vi "LDA_Align_PN_orig.vi"(1 "Align Probe Using":enum16{"Green Beams", "Blue Beams"}(ring), 2 "Use Specification Beam Half-Angle":bool) -> (0 "Beam Data":T1={"Vg1 (Green 1 dir. vect.)"=[0.059117350659853476, -0.996541267827751, 0.05840068807144843], "Vg2  (Green 2 dir. vect.)"=[-0.05232536310393669, -0.9971561380468801, -0.054237373935992664], "Vb1 (Blue 1 dir. vect.)"=[-0.052923229613528855, -0.9969242065933935, 0.057803616456121795], "Vb2 (Blue 1 dir. vect.)"=[0.05971521716944564, -0.9967731992812374, -0.05364030232066602], "Porb (Orb XYZ posn. forced coplanar)"=[2201.0738225655555, -1199.3737231995547, 269.758310600838], "Porb (Orb XYZ posn. - allow skew)"=[2200.796256301178, -1199.3740953152687, 270.0329332816893], "Orb posn. uncertainty, +/- dx, dy, dz"=[0.13878313218879157, 0.00018605785703584843, 0.13731134042564008], "Vp (Actual Probe dir. vect)"=[0.003406702197773746, -0.9999920168246164, 0.0020882210543692924], "Yaw (deg)"=89.80480953887573, "Pitch (deg)"=0.11964634006213794, "In-Plane Roll (deg)"=45.305328966424156, "Beam Half Angle (deg)"=4.544091484248422, "B1 Close P11"=[0.0, 0.0, 0.0], "B1 Far P12"=[2158.01, -491.04, 229.28], "B2 Close P22"=[2158.01, -491.04, 229.28], "B2 Far P21"=[2158.01, -491.04, 229.28], "Projected Roll (deg)"=0.0, "Green Velocity Vector"=[0.0, 0.0, 0.0], "Blue Velocity Vector"=[0.0, 0.0, 0.0], "Probe is facing...."="-", "Calculation Method"=""} {"Vp (Actual Probe dir. vect)" format="%#_6f"; "Vg2  (Green 2 dir. vect.)" format="%#_6f"; "Vg1 (Green 1 dir. vect.)" format="%#_6f"})   [LabVIEW 2010]
uses:
  Controls/LDA_Beam_Cluster.ctl
  Controls/Tunnel_Coordinates.ctl
  Controls/User_Specific_mode.ctl
  Gen Trav/Trav_mode.ctl
  Globals/Trav_pos_global.vi
  Globals/LDA_meas_global_1.vi
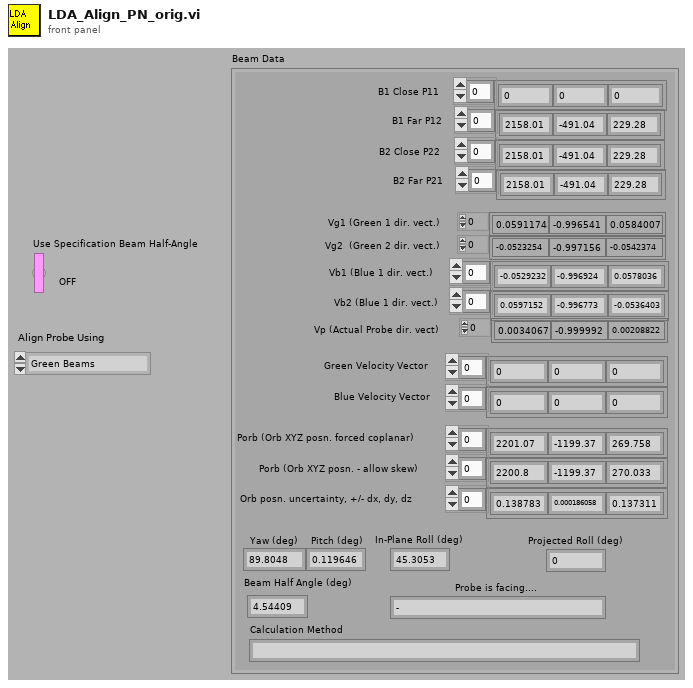
[diagram p1: front panel]
types:
  T1 = typedef "LDA_Beam_Cluster.ctl" = cluster{"Vg1 (Green 1 dir. vect.)":dbl[], "Vg2  (Green 2 dir. vect.)":dbl[], "Vb1 (Blue 1 dir. vect.)":dbl[], "Vb2 (Blue 1 dir. vect.)":dbl[], "Porb (Orb XYZ posn. forced coplanar)":dbl[], "Porb (Orb XYZ posn. - allow skew)":dbl[], "Orb posn. uncertainty, +/- dx, dy, dz":dbl[], "Vp (Actual Probe dir. vect)":dbl[], "Yaw (deg)":dbl, "Pitch (deg)":dbl, "In-Plane Roll (deg)":dbl, "Beam Half Angle (deg)":dbl, "B1 Close P11":dbl[], "B1 Far P12":dbl[], "B2 Close P22":dbl[], "B2 Far P21":dbl[], "Projected Roll (deg)":dbl, "Green Velocity Vector":dbl[], "Blue Velocity Vector":dbl[], "Probe is facing....":string, "Calculation Method":string}
  T2 = typedef "Tunnel_Coordinates.ctl" = enum16{"Work in Tunnel Coordinates", "Work in Model Coordinates"}
  T3 = typedef "User_Specific_mode.ctl" = enum16{"Check VI only", "Run VI"}
  T4 = typedef "Trav_mode.ctl" = enum16{"Move traverse", "Read traverse position", "Teach Position"}
  T5 = enum16{"Load setup from excel file", "Save setup to excel file"}
  T6 = enum16{"Load From Excel File", "Save to Excel File"}
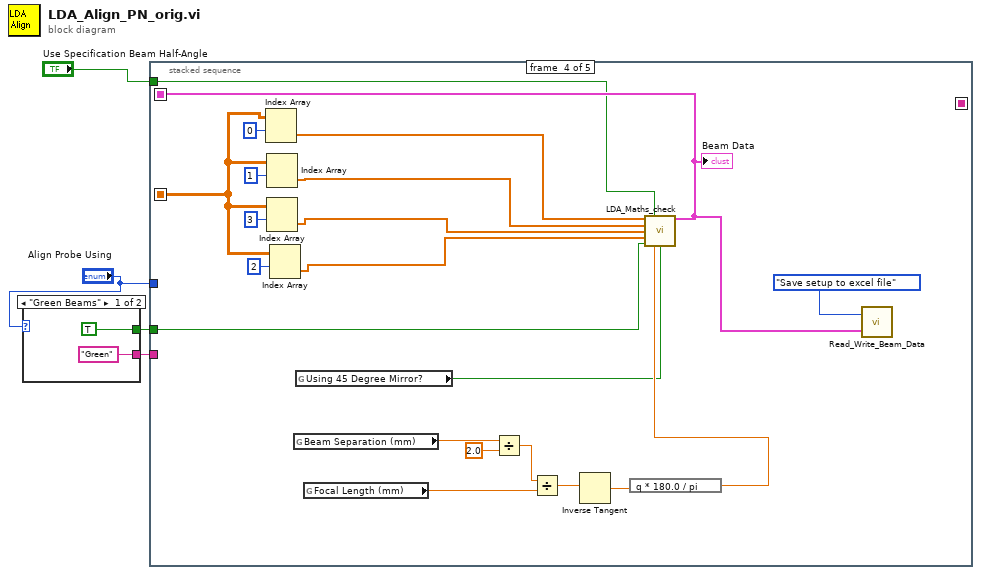
[diagram p0: block diagram]
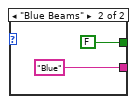
[diagram p2: hidden frame]
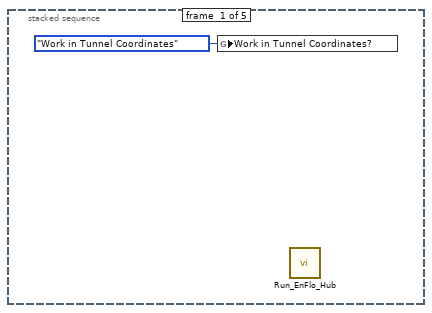
[diagram p3: hidden frame]
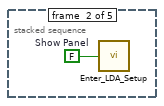
[diagram p4: hidden frame]
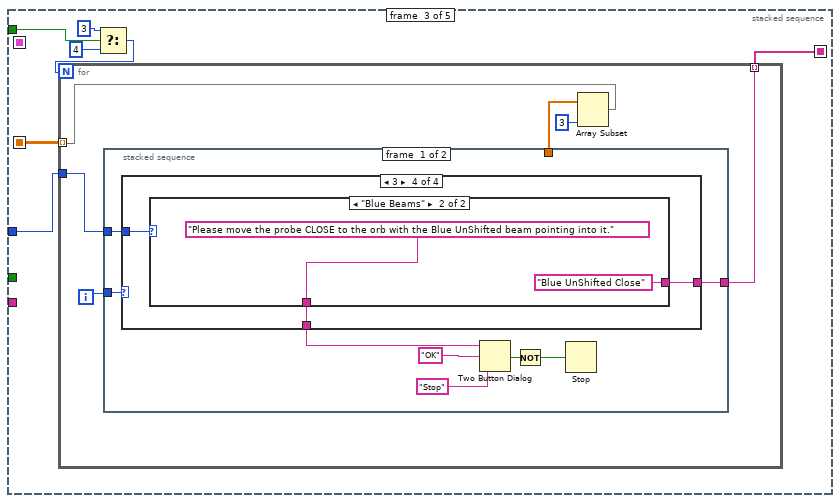
[diagram p5: hidden frame]
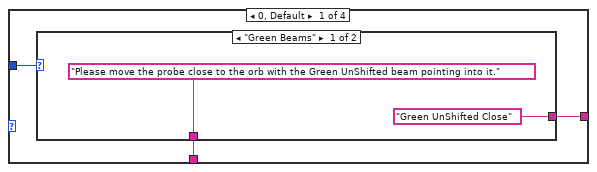
[diagram p6: hidden frame]
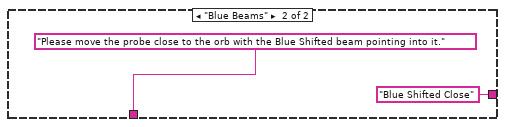
[diagram p7: hidden frame]
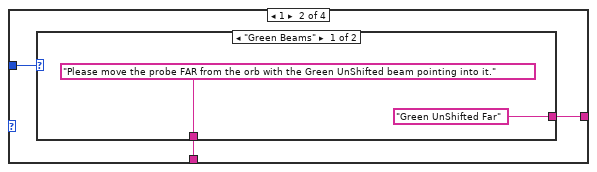
[diagram p8: hidden frame]
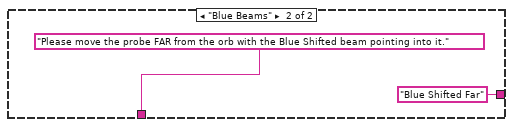
[diagram p9: hidden frame]
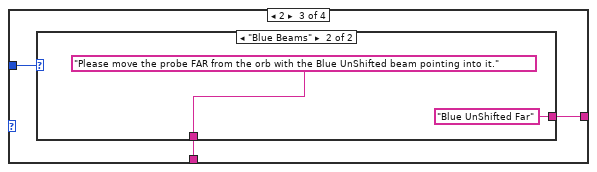
[diagram p10: hidden frame]
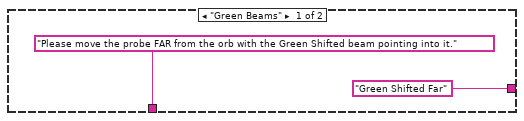
[diagram p11: hidden frame]
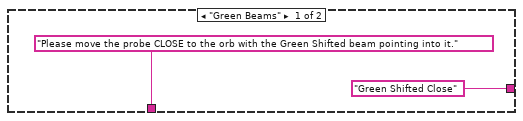
[diagram p12: hidden frame]
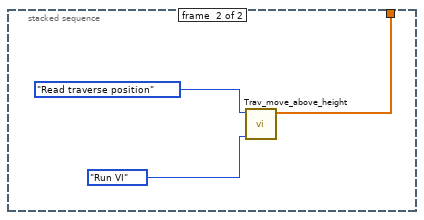
[diagram p13: hidden frame]
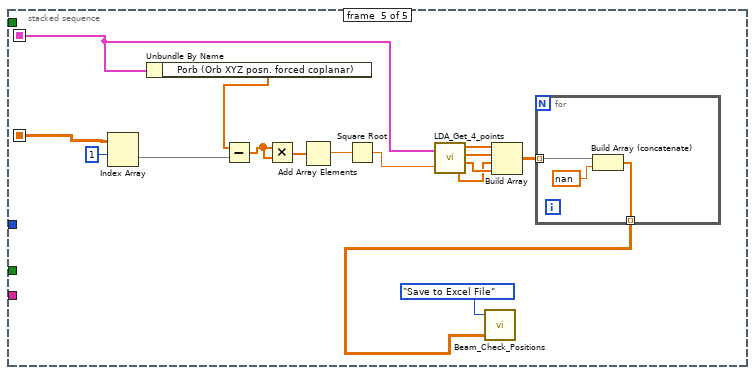
[diagram p14: hidden frame]
diagram:
  n1 = case shown="\"Green Beams\"" "Align Probe Using" {
    tunnel: [TRUE FALSE] -> w4
    tunnel: ["Green" "Blue"] -> w1
    frame "Green Beams" {
    }
    frame "Blue Beams" {
    }
  }
  n2 = stacked-sequence {
    seq-local: [_ _ _ w82 _] -> [_ _ _ _ w95]
    seq-local: [_ _ w11 _ _] -> [_ _ _ w64 w84]
    seq-local: [_ _ w12 _ _] -> [_ _ _ _ _]
    tunnel: w4 -> [_ _ _ w74 _]
    tunnel: "Use Specification Beam Half-Angle" -> [_ _ w16 w73 _]
    tunnel: "Align Probe Using" -> [_ _ w17 _ _]
    tunnel: w1 -> [_ _ _ _ _]
    frame #0 {
      n3 = global write "Trav_pos_global.vi" "Work in Tunnel Coordinates?"(Tunnel_Coordinates."Work in Tunnel Coordinates" ("Work in Tunnel Coordinates?")) -> ()
      n4 = call "Run_EnFlo_Hub.vi"() -> ()  [unwired: 8 in]
    }
    frame #1 {
      w10 = FALSE  # Show Panel
      n5 = call "Enter_LDA_Setup.vi"("Show Panel"=w10) -> ()
    }
    frame #2 {
      n6 = Select(t=3, s=w16, f=4) -> (s? t:f=w13:i32)
      n7 = for {
        N: w13 -> [_]
        tunnel: w17 -> [w23]
        tunnel: [w22] -> w12 mode=indexing
        tunnel: [w18] -> w11 mode=indexing
        i -> [w21]
        n8 = stacked-sequence {
          tunnel: [_ w60] -> w19
          tunnel: w23 -> [w30 _]
          tunnel: [w25 _] -> w22
          tunnel: w21 -> [w24 _]
          frame #0 {
            n9 = case shown="3" w24 {
              tunnel: [w34 w41 w48 w55] -> w31
              tunnel: w30 -> [w33 w40 w47 w54]
              tunnel: [w32 w39 w46 w53] -> w25
              frame 0, Default {
                n10 = case shown="\"Green Beams\"" w33 {
                  tunnel: ["Please move the probe close to the orb with the Green UnShifted beam pointing into it." ("message") "Please move the probe close to the orb with the Blue Shifted beam pointing into it." ("message")] -> w34
                  tunnel: ["Green UnShifted Close" "Blue Shifted Close"] -> w32
                  frame "Green Beams" {
                  }
                  frame "Blue Beams" {
                  }
                }
              }
              frame 1 {
                n11 = case shown="\"Green Beams\"" w40 {
                  tunnel: ["Please move the probe FAR from the orb with the Green UnShifted beam pointing into it." ("message") "Please move the probe FAR from the orb with the Blue Shifted beam pointing into it." ("message")] -> w41
                  tunnel: ["Green UnShifted Far" "Blue Shifted Far"] -> w39
                  frame "Green Beams" {
                  }
                  frame "Blue Beams" {
                  }
                }
              }
              frame 2 {
                n12 = case shown="\"Blue Beams\"" w47 {
                  tunnel: ["Please move the probe FAR from the orb with the Green Shifted beam pointing into it." ("message") "Please move the probe FAR from the orb with the Blue UnShifted beam pointing into it." ("message")] -> w48
                  tunnel: ["Green Shifted Far" "Blue UnShifted Far"] -> w46
                  frame "Green Beams" {
                  }
                  frame "Blue Beams" {
                  }
                }
              }
              frame 3 {
                n13 = case shown="\"Blue Beams\"" w54 {
                  tunnel: ["Please move the probe CLOSE to the orb with the Green Shifted beam pointing into it." ("message") "Please move the probe CLOSE to the orb with the Blue UnShifted beam pointing into it." ("message")] -> w55
                  tunnel: ["Green Shifted Close" "Blue UnShifted Close"] -> w53
                  frame "Green Beams" {
                  }
                  frame "Blue Beams" {
                  }
                }
              }
            }
            n14 = Two Button Dialog(message=w31, 1:"Stop" ("F button name (\"Cancel\")"), 2:"OK" ("T button name (\"OK\")")) -> (T button?=w27:bool)
            n15 = Not(x=w27) -> (.not. x?=w26:bool)
            n16 = Stop(stop? (T)=w26) -> ()
          }
          frame #1 {
            n17 = call "Trav_move_above_height.vi"("Simulate/Run"=User_Specific_mode."Run VI", "Mode"=Trav_mode."Read traverse position") -> ("Trav Position achieved"=w60:dbl[])  [unwired: 8 in, 1 out]
          }
        }
        n18 = Array Subset(array=w19, length=3) -> (w18:dbl[])  [unwired: 1 in]
      }
    }
    frame #3 {
      n19 = Index Array(array=w64, index (row)=0) -> (element=w68:dbl[])  [unwired: 1 in]
      n20 = Index Array(array=w64, index (row)=1) -> (element=w67:dbl[])  [unwired: 1 in]
      n21 = Index Array(array=w64, index (row)=3) -> (element=w66:dbl[])  [unwired: 1 in]
      n22 = Index Array(array=w64, index (row)=2) -> (element=w65:dbl[])  [unwired: 1 in]
      n23 = global read "LDA_meas_global_1.vi" "Beam Separation (mm)"() -> (w81:dbl)
      n24 = global read "LDA_meas_global_1.vi" "Using 45 Degree Mirror?"() -> (w63:bool)
      n25 = global read "LDA_meas_global_1.vi" "Focal Length (mm)"() -> (w78:dbl)
      n26 = Divide(x=w81, y=2.0) -> (x/y=w79:dbl)
      n27 = Divide(x=w79, y=w78) -> (x/y=w76:dbl)
      n28 = Inverse Tangent(1:w76) -> (0:w77:dbl)
      n29 = expression code="q * 180.0 / pi"(w77) -> (w75:dbl)
      n30 = call "LDA_Maths_check.vi"("B1 Close P11"=w68, "Use Specification Beam Half-Angle"=w73, "B1 Far P12"=w67, "B2 Close P22"=w66, "B2 Far P21"=w65, "Use Green Beams (True) or Blue Beams (False)"=w74, "Beam Half-Angle (deg)"=w75, "Using 45 Degree Mirror?"=w63) -> ("Beam Data"=w82:T1)  [unwired: 7 in]
      "Beam Data" <- w82
      n31 = call "Read_Write_Beam_Data.vi"("Beam Data In"=w82, "Mode"=T5."Save setup to excel file") -> ()  [unwired: 1 out]
    }
    frame #4 {
      n32 = Index Array(array=w84, index (row)=1) -> (element=w85:dbl[])  [unwired: 1 in]
      n33 = Unbundle By Name(w95) -> ("Porb (Orb XYZ posn. forced coplanar)"=w99:dbl[])
      n34 = Subtract(x=w99, y=w85) -> (x-y=w98:dbl[])
      n35 = Multiply(x=w98, y=w98) -> (x*y=w97:dbl[])
      n36 = Add Array Elements(numeric array=w97) -> (sum=w96:dbl)
      n37 = Square Root(x=w96) -> (sqrt(x)=w94:dbl)
      n38 = call "LDA_Get_4_points.vi"("Beam Data"=w95, "L, Probe-Normal Distance"=w94) -> ("Pg1"=w93:dbl[], "Pg2"=w92:dbl[], "Pb1"=w88:dbl[], "Pb2"=w87:dbl[])
      n39 = Build Array(w93, w92, w87, w88) -> (w91:dbl[][])
      n40 = for {
        tunnel: w91 -> [w102] mode=indexing
        tunnel: [w100] -> w89 mode=indexing
        n41 = Build Array (concatenate)(w102, nan) -> (w100:dbl[])
      }
      n42 = call "Beam_Check_Positions.vi"("Values"=w89, "Mode"=T6."Save to Excel File") -> ()  [unwired: 1 in, 1 out]
    }
  }
